vi "SUB_COM1_ESC3_ChkDbgMask.vi"(3 "VISA resource name":refnum<visa-resource-name>) -> (0 "MSG OUT":string, 1 "duplicate VISA OUT":refnum<visa-resource-name>)   [LabVIEW 2011]
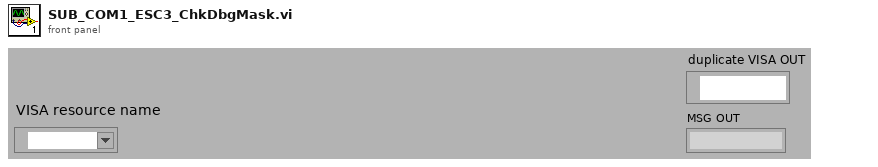
[diagram p1: front panel]
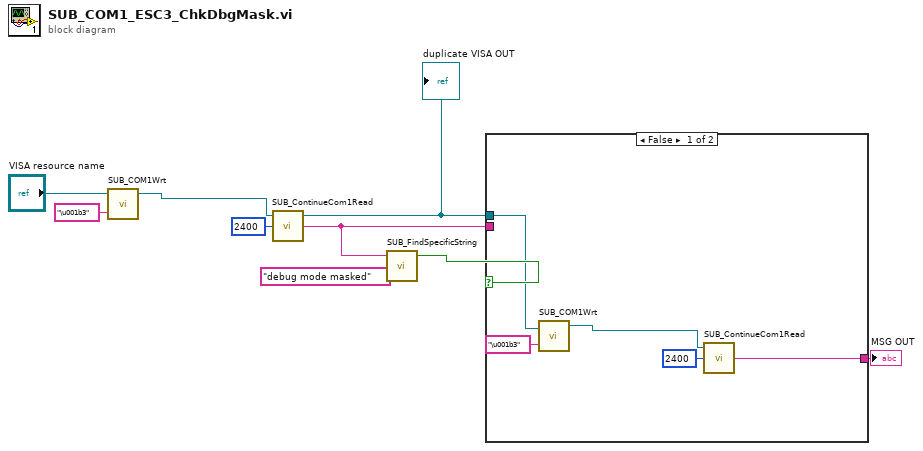
[diagram p0: block diagram]
diagram:
  n1 = call "SUB_COM1Wrt.vi"("VISA resource name"="VISA resource name", "write buffer"="\u001b3") -> ("duplicate VISA resource name"=w8:refnum<visa-resource-name>)  [unwired: 2 out]
  n2 = call "SUB_ContinueCom1Read.vi"("Numeric"=2400, "duplicate VISA resource name 2"=w8) -> ("String"=w2:string, "duplicate VISA resource name"=w4:refnum<visa-resource-name>)  [unwired: 1 in, 1 out]
  "duplicate VISA OUT" <- w4
  n3 = call "SUB_FindSpecificString.vi"("Find this String"="debug mode masked", "String data"=w2) -> ("Found"=w5:bool)  [unwired: 2 in, 1 out]
  n4 = case shown="False" w5 {
    tunnel: w4 -> [w11 _]
    tunnel: [w10 w15] -> w1
    tunnel: w2 -> [_ w15]
    frame False {
      n5 = call "SUB_COM1Wrt.vi"("VISA resource name"=w11, "write buffer"="\u001b3") -> ("duplicate VISA resource name"=w13:refnum<visa-resource-name>)  [unwired: 2 out]
      n6 = call "SUB_ContinueCom1Read.vi"("Numeric"=2400, "duplicate VISA resource name 2"=w13) -> ("String"=w10:string)  [unwired: 1 in, 2 out]
    }
    frame True {
    }
  }
  "MSG OUT" <- w1
